vi "Throw -8717 error.vi"(8 "error in (no error)":errorcluster, 9 "dir speed name":string, 11 "error":bool) -> (0 "error out":errorcluster)   [LabVIEW 2015, in "Engine Simulation Toolkit System Explorer.lvlib"]
uses:
  Engine Simulation Toolkit System Explorer.lvlib
  <vilib>/Utility/error.llb/Error Cluster From Error Code.vi
  <vilib>/ErrorRing/Error Ring.xnode
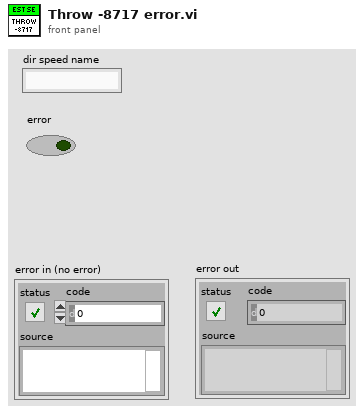
[diagram p1: front panel]
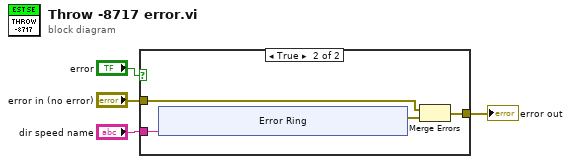
[diagram p0: block diagram]
diagram:
  n1 = case shown="True" "error" {
    tunnel: "error in (no error)" -> [w5 w9]
    tunnel: [w5 w7] -> w4
    tunnel: "dir speed name" -> [_ w6]
    frame False {
    }
    frame True {
      n2 = xnode "Error Ring"("parameter 0"=w6) -> ("error out"=w8:errorcluster)
      n3 = Merge Errors(w9, w8) -> (w7:errorcluster)
    }
  }
  "error out" <- w4
